vi "Change State.vi"(8 "error in (no error)":errorcluster, 10 "Target State":refnum<class "_State Machine Actor.lvclass">, 11 "_State Machine Actor in":refnum<class "_State Machine Actor.lvclass">) -> (0 "error out":errorcluster, 3 "_State Machine Actor out":refnum<class "_State Machine Actor.lvclass">)   [LabVIEW 2024]
uses:
  _State Machine Actor.lvclass
  _State Machine Actor.lvclass/_State Machine Actor.ctl
  C:/Program Files (x86)/National Instruments/LabVIEW 2024/vi.lib/ActorFramework/Actor/Actor.lvclass
  C:/Users/uspoaotto/OneDrive - Oregon Tool/Desktop/working copies/stateMachineActor/src/_State Machine Actor/_State Machine Actor/_State Machine Actor.lvclass
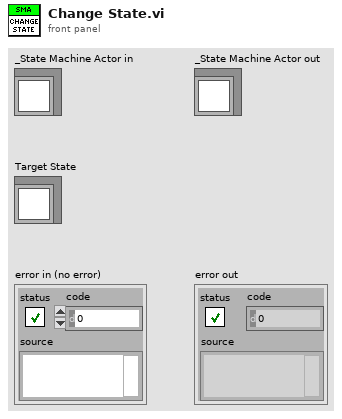
[diagram p1: front panel]
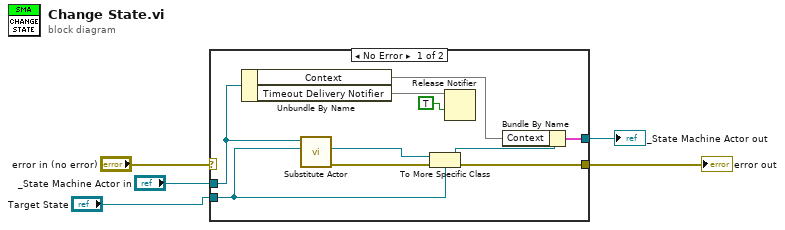
[diagram p0: block diagram]
diagram:
  n1 = case shown="No Error" "error in (no error)" {
    selector: "error in (no error)" -> [_ w17]
    tunnel: [w8 w17] -> w4
    tunnel: [w10 w16] -> w2
    tunnel: "_State Machine Actor in" -> [w12 w16]
    tunnel: "Target State" -> [w14 _]
    frame No Error {
      n2 = Unbundle By Name(w12) -> ("Context"=w11, "Timeout Delivery Notifier"=w7)
      n3 = call-dynamic "Substitute Actor.vi"("Substitute Actor in"=w14, "Current Actor"=w12) -> ("error out"=w9:errorcluster, "Substitute Actor out"=w15:refnum<class "Actor.lvclass">)  [unwired: 8 in]
      n4 = To More Specific Class(target class=w14, reference=w15, error in=w9) -> (specific class reference=w13:refnum<class "_State Machine Actor.lvclass">, error out=w8:errorcluster)
      n5 = Release Notifier(notifier=w7, force destroy? (F)=TRUE) -> ()  [unwired: 1 in, 3 out]
      n6 = Bundle By Name(cluster=w13, "Context"=w11) -> (w10:cluster{})
    }
    frame Error {
    }
  }
  "error out" <- w4
  "_State Machine Actor out" <- w2
